vi "test_Series cRIO PWM CAN Temp.vi"(8 "Error In":errorcluster) -> (0 "Error Out":errorcluster)   [LabVIEW 2023]
uses:
  DIO/DO DAQmx Fixed Freq PWM CFG/DO DAQmx Fixed Freq PWM CFG.lvclass
  Devices/NEO480HTA/Real All CFG/Read All CFG.lvclass
  Series/Series Base/Series Base.lvclass
  <vilib>/ActorFramework/Actor/Actor.lvclass
  <vilib>/ActorFramework/Stop Msg/Stop Msg.lvclass
  Sample Tasks/Sample Airtemp PWM Control/Sample Airtemp PWM Control.lvclass
  Study/Study Actor/Study Actor/Study Actor.lvclass
  Series/Series Actor/Series Actor/Series Actor.lvclass
  Series/ISeries Actor/ISeries Actor Messages/Start Tasks Msg/Start Tasks Msg.lvclass
  DIO/Virtual DIO/Virt PWM Fixed Freq Generator/Virt DAQmx Fixed Freq PWM Generator.lvclass
panel:
  in  "Start Series Button":bool
  in  "Kill Series Actor Button":bool
  out "Temperature Chart Lossy":dbl(graph)
  in  "Temp Setpoint":dbl=23.0 format="%#_g °C"
  in  "stop":bool
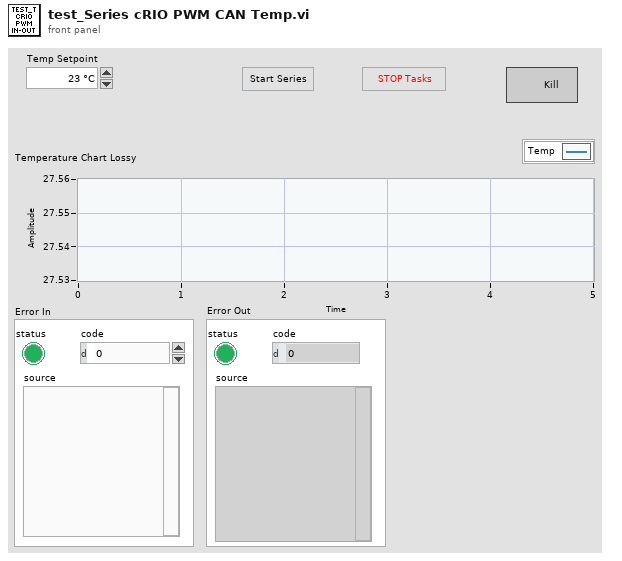
[diagram p1: front panel]
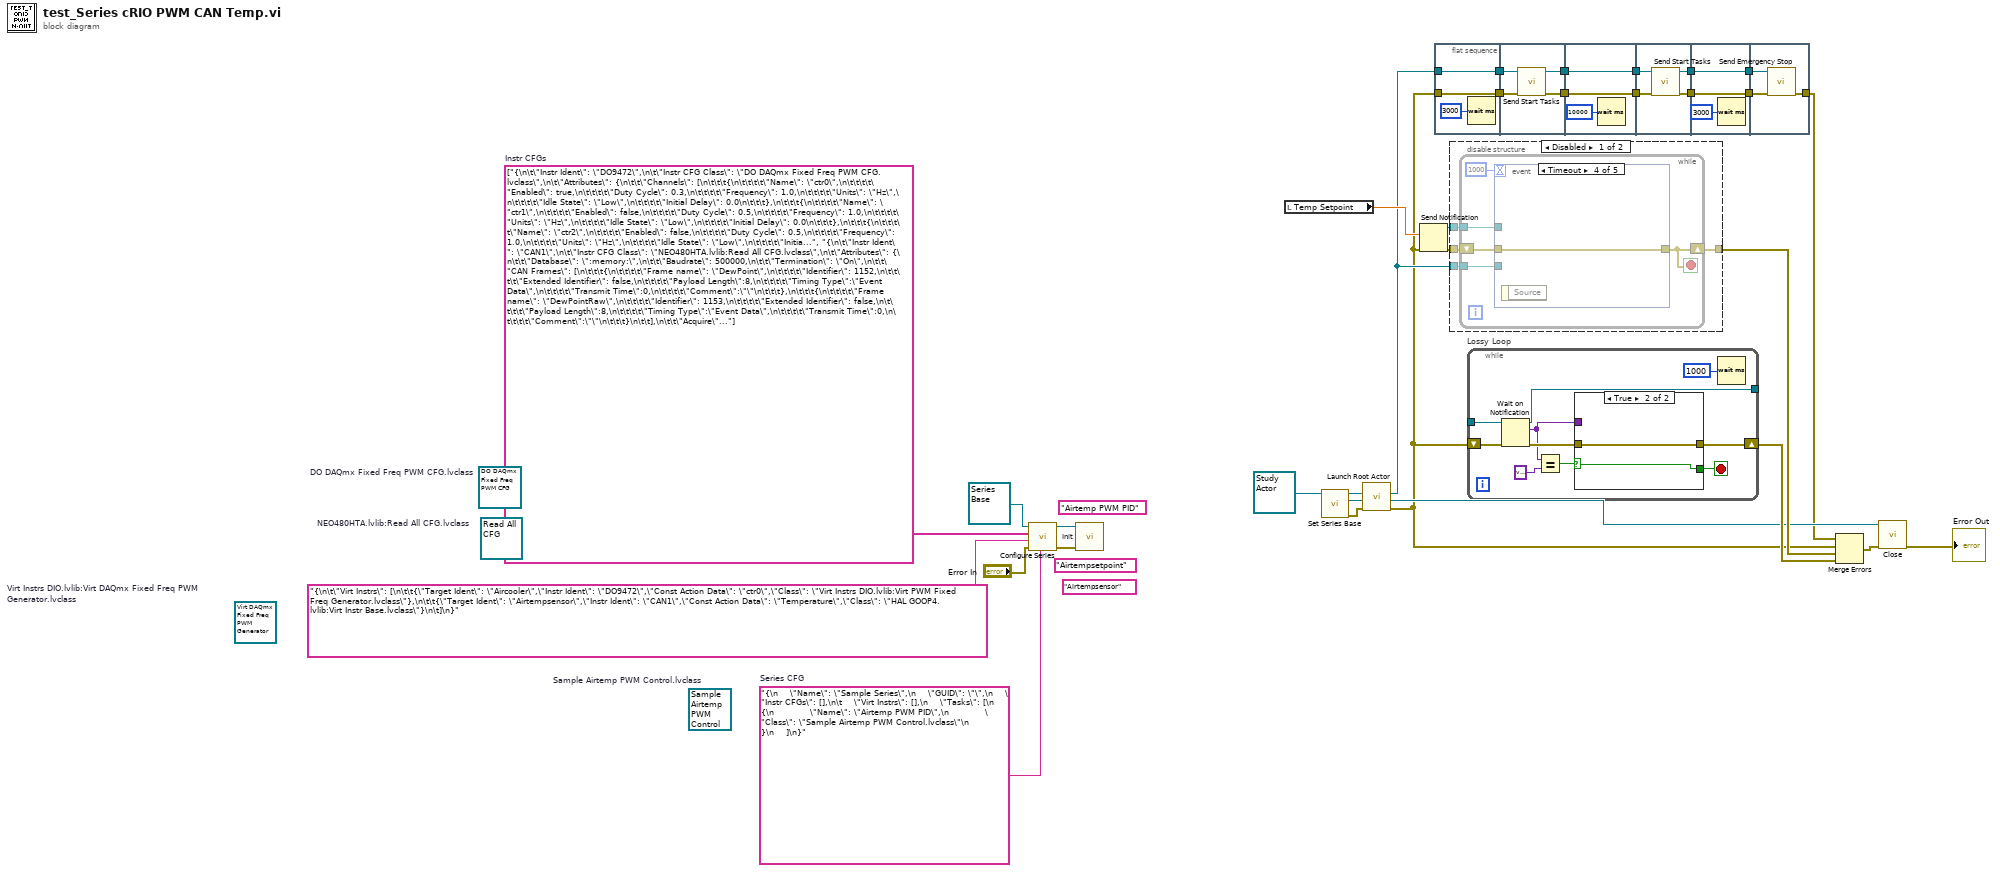
[diagram p0: block diagram]
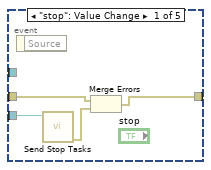
[diagram p2: hidden frame]
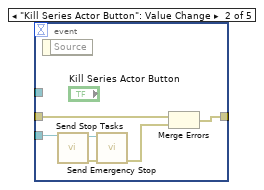
[diagram p3: hidden frame]
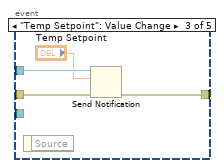
[diagram p4: hidden frame]
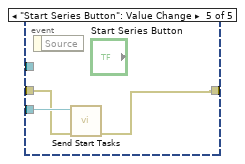
[diagram p5: hidden frame]
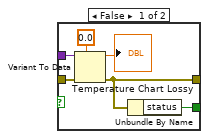
[diagram p7: hidden frame]
diagram:
  (unwired) refnum<class "Sample Airtemp PWM Control.lvclass"> refnum  # Sample Airtemp PWM Control.lvclass
  w22 = "Airtempsensor" ("Target Name")
  w21 = "Airtemp PWM PID"
  w25 = "Airtempsetpoint" ("Name")
  (unwired) refnum<class "Virt DAQmx Fixed Freq PWM Generator.lvclass"> refnum  # Virt Instrs DIO.lvlib:Virt DAQmx Fixed Freq PWM Generator.lvclass
  w36 = "{\n    \"Name\": \"Sample Series\",\n    \"GUID\": \"\",\n    \"Instr CFGs\": [],\n\t    \"Virt Instrs\": [],\n    \"Tasks\": [\n        {\n            \"Name\": \"Airtemp PWM PID\",\n            \"Class\": \"Sample Airtemp PWM Control.lvclass\"\n        }\n    ]\n}"  # Series CFG
  (unwired) refnum<class "Read All CFG.lvclass"> refnum  # NEO480HTA.lvlib:Read All CFG.lvclass
  (unwired) refnum<class "DO DAQmx Fixed Freq PWM CFG.lvclass"> refnum  # DO DAQmx Fixed Freq PWM CFG.lvclass
  w34 = string[] ["{\n\t\"Instr Ident\": \"DO9472\",\n\t\"Instr CFG Class\": \"DO DAQmx Fixed Freq PWM CFG.lvclass\",\n\t\"Attributes\": {\n\t\t\"Channels\": [\n\t\t\t{\n\t\t\t\t\"Name\": \"ctr0\",\n\t\t\t\t\"Enabled\": true,\n\t\t\t\t\"Duty Cycle\": 0.3,\n\t\t\t\t\"Frequency\": 1.0,\n\t\t\t\t\"Units\": \"Hz\",\n\t\t\t\t\"Idle State\": \"Low\",\n\t\t\t\t\"Initial Delay\": 0.0\n\t\t\t},\n\t\t\t{\n\t\t\t\t\"Name\": \"ctr1\",\n\t\t\t\t\"Enabled\": false,\n\t\t\t\t\"Duty Cycle\": 0.5,\n\t\t\t\t\"Frequency\": 1.0,\n\t\t\t\t\"Units\": \"Hz\",\n\t\t\t\t\"Idle State\": \"Low\",\n\t\t\t\t\"Initial Delay\": 0.0\n\t\t\t},\n\t\t\t{\n\t\t\t\t\"Name\": \"ctr2\",\n\t\t\t\t\"Enabled\": false,\n\t\t\t\t\"Duty Cycle\": 0.5,\n\t\t\t\t\"Frequency\": 1.0,\n\t\t\t\t\"Units\": \"Hz\",\n\t\t\t\t\"Idle State\": \"Low\",\n\t\t\t\t\"Initial Delay\": 0.0\n\t\t\t},\n\t\t\t{\n\t\t\t\t\"Name\": \"ctr3\",\n\t\t\t\t\"Enabled\": false,\n\t\t\t\t\"Duty Cycle\": 0.5,\n\t\t\t\t\"Frequency\": 1.0,\n\t\t\t\t\"Units\": \"Hz\",\n\t\t\t\t\"Idle State\": \"Low\",\n\t\t\t\t\"Initial Delay\": 0.0\n\t\t\t}\n\t\t],\n\t\t\"Timing\": {\n\t\t\t\"Samples per Channel\": 1000,\n\t\t\t\"Sample Mode\": \"Continuous Samples\",\n\t\t\t\"Sample Rate\": 0.0,\n\t\t\t\"Sample Clock Source\": \"Implicit\",\n\t\t\t\"Active Edge\": \"Rising\"\n\t\t},\n\t\t\"Trigger\": {\n\t\t\t\"Trigger Type\": \"No Trigger\"\n\t\t}\n\t}\n}", "{\n\t\"Instr Ident\": \"CAN1\",\n\t\"Instr CFG Class\": \"NEO480HTA.lvlib:Read All CFG.lvclass\",\n\t\"Attributes\": {\n\t\t\"Database\": \":memory:\",\n\t\t\"Baudrate\": 500000,\n\t\t\"Termination\": \"On\",\n\t\t\"CAN Frames\": [\n\t\t\t{\n\t\t\t\t\"Frame name\": \"DewPoint\",\n\t\t\t\t\"Identifier\": 1152,\n\t\t\t\t\"Extended Identifier\": false,\n\t\t\t\t\"Payload Length\":8,\n\t\t\t\t\"Timing Type\":\"Event Data\",\n\t\t\t\t\"Transmit Time\":0,\n\t\t\t\t\"Comment\":\"\"\n\t\t\t},\n\t\t\t{\n\t\t\t\t\"Frame name\": \"DewPointRaw\",\n\t\t\t\t\"Identifier\": 1153,\n\t\t\t\t\"Extended Identifier\": false,\n\t\t\t\t\"Payload Length\":8,\n\t\t\t\t\"Timing Type\":\"Event Data\",\n\t\t\t\t\"Transmit Time\":0,\n\t\t\t\t\"Comment\":\"\"\n\t\t\t}\n\t\t],\n\t\t\"Acquire\": {\n\t\t\t\"Type\": \"Read Frame\"\n\t\t}\n\t}\n}"]  # Instr CFGs
  n1 = call "Configure Series.vi"("Series CFG"=w36, "error in (no error)"="Error In", "Virt Instrs CFG"="{\n\t\"Virt Instrs\": [\n\t\t{\"Target Ident\": \"Aircooler\",\"Instr Ident\": \"DO9472\",\"Const Action Data\": \"ctr0\",\"Class\": \"Virt Instrs DIO.lvlib:Virt PWM Fixed Freq Generator.lvclass\"},\n\t\t{\"Target Ident\": \"Airtempsensor\",\"Instr Ident\": \"CAN1\",\"Const Action Data\": \"Temperature\",\"Class\": \"HAL GOOP4.lvlib:Virt Instr Base.lvclass\"}\n\t]\n}", "Instr CFGs"=w34, "HAL GOOP4:Series Base in"=refnum<class "Series Base.lvclass"> refnum ("HAL GOOP4.lvlib:Study Base.lvclass")) -> ("error out"=w38:errorcluster, "HAL GOOP4:Series Base out"=w39:refnum<class "Series Base.lvclass">)  [unwired: 5 in]
  n2 = call-dynamic "Init.vi"("error in"=w38, "HAL GOOP4:Series Base in"=w39) -> ("error out"=w32:errorcluster, "HAL GOOP4:Series Base out"=w28:refnum<class "Series Base.lvclass">)  [unwired: 8 in]
  n3 = local read "Temp Setpoint"() -> (w29:dbl)
  n4 = call "Set Series Base.vi"("Series Actor in"=refnum<class "Study Actor.lvclass"> refnum ("HAL GOOP4.lvlib:Study Actor.lvlib:Study Actor.lvclass")) -> ("error out"=w27:errorcluster, "Series Actor out"=w26:refnum<class "Series Actor.lvclass">, "error in (no error)"=w23:errorcluster, "Series Base"=w14:refnum<class "Series Base.lvclass">)  [unwired: 7 in]
  n5 = call <vilib>:"Launch Root Actor.vi"("error in (no error)"=w27, "Actor"=w26) -> ("error out"=w12:errorcluster, "Actor's Enqueuer"=w13:refnum<class "Message Enqueuer.lvclass">)  [unwired: 8 in]
  n6 = Send Notification(notification=w29, error in (no error)=w12) -> (notifier=w19:refnum<notifier>, notifier out=w18:refnum<notifier>, error out=w30:errorcluster)
  n7 = flat-sequence {
    tunnel: w12 -> [w41]
    tunnel: w13 -> [w42]
    tunnel: [w42] -> w11
    tunnel: [w41] -> w10
    tunnel: w11 -> [w46]
    tunnel: w10 -> [w45]
    tunnel: [w44] -> w9
    tunnel: [w43] -> w8
    tunnel: w9 -> [w48]
    tunnel: w8 -> [w47]
    tunnel: [w48] -> w7
    tunnel: [w47] -> w6
    tunnel: w7 -> [w52]
    tunnel: w6 -> [w53]
    tunnel: [w51] -> w4
    tunnel: [w50] -> w2
    tunnel: [w55] -> w5
    tunnel: w4 -> [w55]
    tunnel: [w54] -> w3
    tunnel: w2 -> [w54]
    tunnel: w5 -> [w58]
    tunnel: w3 -> [w59]
    tunnel: [w57] -> w1
    frame #0 {
      n8 = Wait (ms)(milliseconds to wait=u32 3000) -> ()  [unwired: 1 out]
    }
    frame #1 {
      n9 = call "Send Start Tasks.vi"("error in (no error)"=w45, "Message Enqueuer"=w46) -> ("error out"=w43:errorcluster, "Message Enqueuer out"=w44:refnum<class "Message Enqueuer.lvclass">)  [unwired: 8 in]
    }
    frame #2 {
      n10 = Wait (ms)(milliseconds to wait=u32 10000) -> ()  [unwired: 1 out]
    }
    frame #3 {
      n11 = call "Send Start Tasks.vi"("error in (no error)"=w53, "Message Enqueuer"=w52) -> ("error out"=w50:errorcluster, "Message Enqueuer out"=w51:refnum<class "Message Enqueuer.lvclass">)  [unwired: 8 in]
    }
    frame #4 {
      n12 = Wait (ms)(milliseconds to wait=u32 3000) -> ()  [unwired: 1 out]
    }
    frame #5 {
      n13 = call <vilib>:"Send Emergency Stop.vi"("error in (no error)"=w59, "Message Enqueuer"=w58) -> ("error out"=w57:errorcluster)  [unwired: 9 in]
    }
  }
  n14 = disable-structure shown="Disabled" {
    disable-tunnel: w30 -> [w63 _]
    disable-tunnel: w18 -> [w62 _]
    disable-tunnel: [w61 _] -> w15
    disable-tunnel: w13 -> [w60 _]
    frame Disabled {
      n15 = while {
        shift-right: [w68] -> w61
        shift-left: w63 -> [w67]
        tunnel: w60 -> [w66]
        tunnel: w62 -> [w65]
        stop <- w68 stop-if-true
        n16 = event shown="[3] Timeout" {
          selector: _ -> [_ _ _ _ _]
          dyn-events: _ -> [_ _ _ _ _]
          timeout: 1000 -> [_ _ _ _ _]
          tunnel: [w69 w76 w80 w83 w84] -> w68
          tunnel: w65 -> [_ _ w82 _ _]
          tunnel: w67 -> [w70 w75 w79 w83 w85]
          tunnel: w66 -> [w72 w78 _ _ w86]
          event "stop": Value Change {
            n17 = event-data() -> ()  [unwired: 1 in, 1 out]
            n18 = call "Send Stop Tasks.vi"("Message Enqueuer"=w72) -> ("error out"=w71:errorcluster)  [unwired: 9 in, 1 out]
            n19 = Merge Errors(w70, w71) -> (w69:errorcluster)
          }
          event "Kill Series Actor Button": Value Change {
            n20 = event-data() -> ()  [unwired: 1 in, 1 out]
            n21 = call "Send Stop Tasks.vi"("Message Enqueuer"=w78) -> ("error out"=w77:errorcluster, "Message Enqueuer out"=w73:refnum<class "Message Enqueuer.lvclass">)  [unwired: 9 in]
            n22 = call <vilib>:"Send Emergency Stop.vi"("error in (no error)"=w77, "Message Enqueuer"=w73) -> ("error out"=w74:errorcluster)  [unwired: 9 in]
            n23 = Merge Errors(w75, w74) -> (w76:errorcluster)
          }
          event "Temp Setpoint": Value Change {
            n24 = event-data() -> ()  [unwired: 1 in, 1 out]
            n25 = Send Notification(notification="Temp Setpoint", notifier=w82, error in (no error)=w79) -> (error out=w80:errorcluster)  [unwired: 1 out]
          }
          event Timeout {
            n26 = event-data() -> ()  [unwired: 1 in, 1 out]
          }
          event "Start Series Button": Value Change {
            n27 = event-data() -> ()  [unwired: 1 in, 1 out]
            n28 = call "Send Start Tasks.vi"("error in (no error)"=w85, "Message Enqueuer"=w86) -> ("error out"=w84:errorcluster)  [unwired: 8 in, 1 out]
          }
        }
      }
    }
    frame Enabled {
    }
  }
  n29 = while "Lossy Loop" {
    tunnel: [w92] -> w20
    shift-right: [w93] -> w16
    shift-left: w12 -> [w94]
    tunnel: [w91] -> _
    stop <- w90 stop-if-true
    n30 = Wait on Notification(notifier=w92, error in (no error)=w94) -> (notifier out=w91:refnum<notifier>, notification=w88:variant, error out=w96:errorcluster)  [unwired: 2 in, 1 out]
    n31 = Equal?(x=w88, y=variant) -> (x = y?=w87:bool)
    n32 = case shown="True" w87 {
      selector: w87 -> [_ w104]
      tunnel: w96 -> [w102 w103]
      tunnel: [w100 w103] -> w93
      tunnel: [w97 w104] -> w90
      tunnel: w88 -> [w98 _]
      frame False {
        n33 = Variant To Data(error in=w102, type=0.0 ("Waveform"), Variant=w98) -> (data=→"Temperature Chart Lossy":dbl, error out=w100:errorcluster)
        n34 = Unbundle By Name(w100) -> ("status"=w97:bool)
      }
      frame True {
      }
    }
    n35 = Wait (ms)(milliseconds to wait=u32 1000) -> ()  [unwired: 1 out]
  }
  n36 = Merge Errors(w1, w12, w15, w16) -> (w17:errorcluster)
  n37 = call-dynamic "Close.vi"("error in"=w17, "Series Base in"=w14) -> ("error out"=→"Error Out":errorcluster)  [unwired: 8 in, 1 out]
